vi "DefBallTrajSkill.vi"(8 "error in (no error)":errorcluster, 9 "Robot":refnum<class "Robot.lvclass">, 10 "Game":refnum<class "Game.lvclass">, 11 "DefBallTrajSkill in":refnum<class "DefBallTrajSkill.lvclass">) -> (0 "error out":errorcluster, 2 "robot out":refnum<class "Robot.lvclass">, 3 "DefBallTrajSkill out":refnum<class "DefBallTrajSkill.lvclass">)   [LabVIEW 2023, in "DefBallTrajSkill.lvclass"]
uses:
  DefBallTrajSkill.lvclass
  Game_class/Game.lvclass
  Robot_class/Robot.lvclass
  Game_class/Game.lvclass/Game.ctl
  Object_class/Object.lvclass/Object.ctl
  Ball_class/Ball.lvclass/Ball.ctl
  Parameters_class/Parameters.lvclass/Parameters.ctl
  Utilities_class/Utilities.lvclass
  Robot_class/Robot.lvclass/Robot.ctl
  Game_class/Read BallRef.vi
  Game_class/Read FieldRef.vi
  Game_class/Read Parameters.lvclass.vi
  Parameters_class/Read GoalieInFrontGoal.vi
  Object_class/Read x.vi
  Object_class/Read y.vi
  Ball_class/Read v_x.vi
  Ball_class/Read v_y.vi
  Robot_class/Write dest_x.vi
  Robot_class/Write dest_y.vi
  Robot_class/Write dest_orientation.vi
  Ball_class/Ball.lvclass
  C:/Users/roboi/Downloads/VSS_AI-Larc2023 - Copia (2)/Object_class/Object.lvclass
  Field_class/Field.lvclass
  Parameters_class/Parameters.lvclass
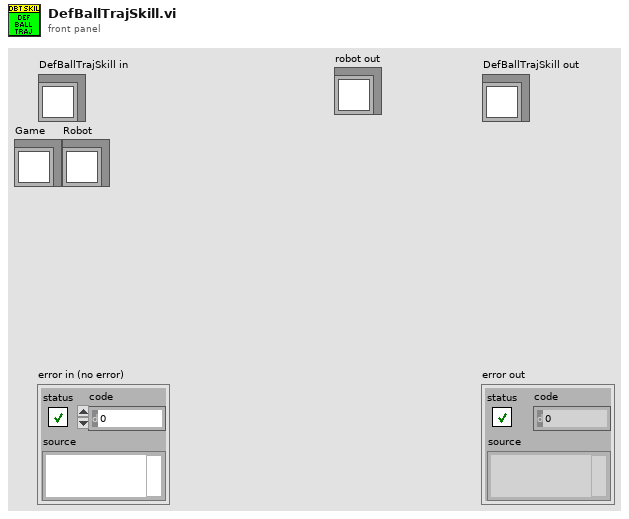
[diagram p1: front panel]
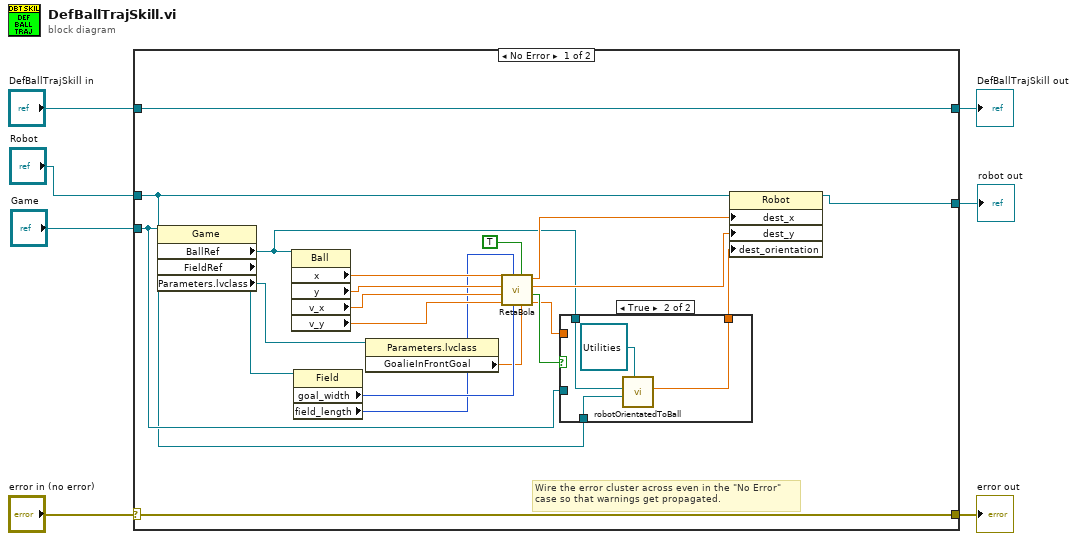
[diagram p0: block diagram]
diagram:
  n1 = case shown="No Error" "error in (no error)" {
    selector: "error in (no error)" -> [w27 w35]
    tunnel: [w27 w35] -> w6
    tunnel: [w28 w34] -> w4
    tunnel: "DefBallTrajSkill in" -> [w28 w34]
    tunnel: "Game" -> [w12 _]
    tunnel: "Robot" -> [w11 _]
    tunnel: [w16 _] -> w1
    frame No Error {
      # "Wire the error cluster across even in the \"No Error\"\ncase so that warnings get propagated."
      n2 = property class="Game"(reference=w12) -> ("BallRef"=w8:refnum<class "Ball.lvclass">, "FieldRef"=w22:refnum<class "Field.lvclass">, "Parameters.lvclass"=w10:refnum<class "Parameters.lvclass">)  [unwired: 1 in, 2 out]
      n3 = property class="Ball"(reference=w8) -> ("x"=w26:dbl, "y"=w25:dbl, "v_x"=w24:dbl, "v_y"=w23:dbl)  [unwired: 1 in, 2 out]
      n4 = property class="Field"(reference=w22) -> ("goal_width"=w21:i32, "field_length"=w20:i32)  [unwired: 1 in, 2 out]
      n5 = property class="Parameters.lvclass"(reference=w10) -> ("GoalieInFrontGoal"=w9:dbl)  [unwired: 1 in, 2 out]
      n6 = call "RetaBola.vi"("DistInFrontGoal"=w9, "Meio?"=TRUE, "Goal Width"=w21, "Field Lenght"=w20, "Vy bola"=w23, "Vx bola"=w24, "Y bola"=w25, "X bola"=w26) -> ("Orientação"=w13:dbl, "Low ball velocity?"=w15:bool, "Y goleiro"=w17:dbl, "X goleiro"=w18:dbl)
      n7 = case shown="True" w15 {
        tunnel: [w29 w32] -> w14
        tunnel: w13 -> [w29 _]
        tunnel: w12 -> [_ _]
        tunnel: w11 -> [_ w31]
        tunnel: w8 -> [_ w30]
        frame False {
        }
        frame True {
          n8 = call "robotOrientatedToBall.vi"("Robot"=w31, "BallRef"=w30, "Utilities in"=refnum<class "Utilities.lvclass"> refnum) -> ("Orientation"=w32:dbl)  [unwired: 6 in, 2 out]
        }
      }
      n9 = property class="Robot"(reference=w11, "dest_x"=w18, "dest_y"=w17, "dest_orientation"=w14) -> (reference out=w16:refnum<class "Robot.lvclass">)  [unwired: 1 in, 1 out]
    }
    frame Error {
    }
  }
  "error out" <- w6
  "DefBallTrajSkill out" <- w4
  "robot out" <- w1
